vi "CH_LM Revision Query.vi"(0 "Meter Index":i32, 5 "error in (no error)":errorcluster, 7 "Timeout / ms (3000)":i32=3000, 9 "Lock Timeout / ms (1000)":i32=1000) -> (10 "Module":string, 11 "Lock timed out":bool, 12 "Vendor":string, 14 "Meter Index":i32, 15 "Instrument Driver Revision":string, 17 "Instrument Firmware Revision":string, 18 "Instrument Firmware Date":string, 19 "error out":errorcluster)   [LabVIEW 2012, in "CH_LM.lvlib"]
doc: "Queries the current instrument firmware revision and instrument driver revision.\n\nRefer to the Readme file for detailed driver information including modification history."
uses:
  CH_LM.lvlib
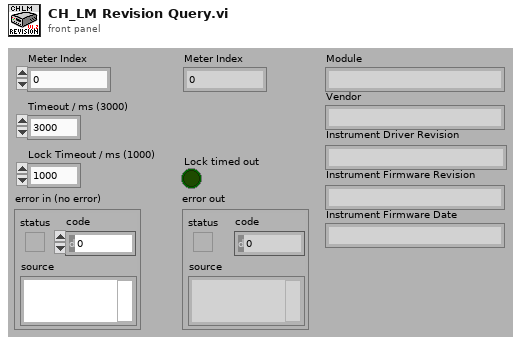
[diagram p1: front panel]
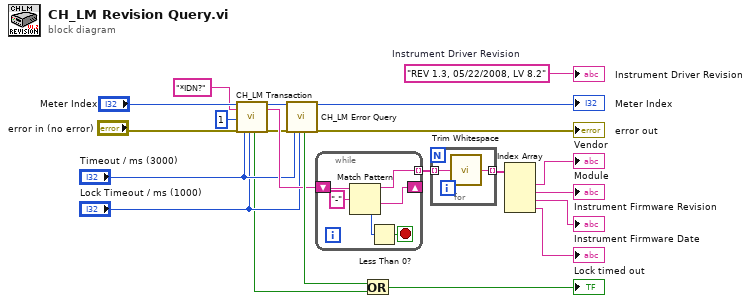
[diagram p0: block diagram]
diagram:
  w21 = "REV 1.3, 05/22/2008, LV 8.2"  # Instrument Driver Revision
  n1 = call "CH_LM Transaction.vi"("Meter Index"="Meter Index", "Command String"="*IDN?", "NofStrings (-1:all)"=1, "error in (no error)"="error in (no error)", "Timeout / ms (3000)"="Timeout / ms (3000)", "Lock Timeout / ms (1000)"="Lock Timeout / ms (1000)") -> ("Lock timed out"=w1:bool, "Meter Index"=w6:i32, "Response"=w5:string, "error out"=w4:errorcluster)  [unwired: 10 out]
  n2 = call "CH_LM Error Query.vi"("Meter Index"=w6, "error in (no error)"=w4, "Timeout / ms (3000)"="Timeout / ms (3000)", "Lock Timeout / ms (1000)"="Lock Timeout / ms (1000)") -> ("Lock timed out"=w12:bool, "Meter Index"=→"Meter Index":i32, "error out"=→"error out":errorcluster)  [unwired: 13 out]
  n3 = while {
    shift-right: [w26] -> _
    shift-left: w5 -> [w27]
    tunnel: [w25] -> w20 mode=indexing
    stop <- w23 stop-if-true
    n4 = Match Pattern(string=w27, regular expression="-") -> (before substring=w25:string, after substring=w26:string, offset past match=w24:i32)  [unwired: 2 out]
    n5 = Less Than 0?(x=w24) -> (x < 0?=w23:bool)
  }
  n6 = Or(x=w12, y=w1) -> (x .or. y?=→"Lock timed out":bool)
  n7 = for {
    tunnel: w20 -> [w29] mode=indexing
    tunnel: [w28] -> w19 mode=indexing
    n8 = call <vilib>:"Trim Whitespace.vi"("string"=w29) -> ("trimmed string"=w28:string)  [unwired: 1 in]
  }
  n9 = Index Array(array=w19) -> (element #1=→"Vendor":string, element #2=→"Module":string, element #3=→"Instrument Firmware Revision":string, element #4=→"Instrument Firmware Date":string)  [unwired: 4 in]
  "Instrument Driver Revision" <- w21
